vi "initUndo_Redo_stacks.vi"(8 "error in (no error)":errorcluster, 11 "ScriptEditorV2 in":refnum<class "ScriptEditorV2.lvclass">) -> (0 "error out":errorcluster, 3 "ScriptEditorV2 out":refnum<class "ScriptEditorV2.lvclass">)   [LabVIEW 2009, in "Views.lvlib" / "ScriptEditor.lvlib" / "ScriptEditorV2.lvclass"]
uses:
  ScriptEditorV2.lvclass
  ScriptEditorV2.lvclass/ScriptEditorV2.ctl
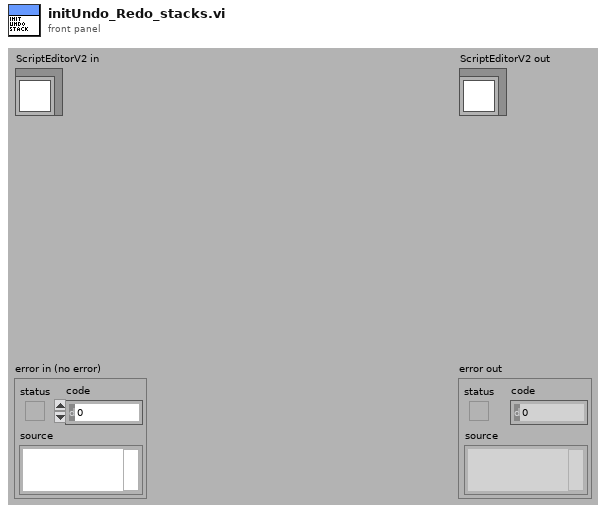
[diagram p1: front panel]
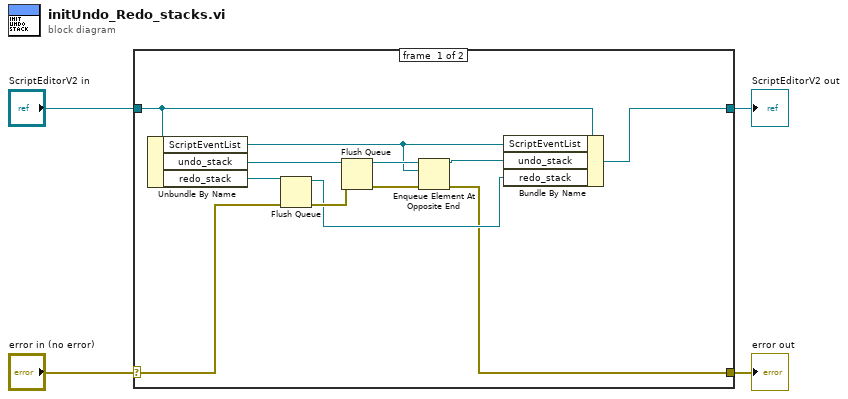
[diagram p0: block diagram]
diagram:
  n1 = case shown="No Error" "error in (no error)" {
    selector: "error in (no error)" -> [w13 w18]
    tunnel: [w5 w18] -> w3
    tunnel: [w6 w17] -> w1
    tunnel: "ScriptEditorV2 in" -> [w7 w17]
    frame #0 {
      n2 = Unbundle By Name(w7) -> ("ScriptEventList"=w10:refnum<class "ScriptEventList.lvclass">, "undo_stack"=w16:refnum<queue>, "redo_stack"=w14:refnum<queue>)
      n3 = Flush Queue(queue=w14, error in (no error)=w13) -> (queue out=w8:refnum<queue>, error out=w15:errorcluster)  [unwired: 1 out]
      n4 = Flush Queue(queue=w16, error in (no error)=w15) -> (queue out=w12:refnum<queue>, error out=w11:errorcluster)  [unwired: 1 out]
      n5 = Enqueue Element At Opposite End(queue=w12, element=w10, error in (no error)=w11) -> (queue out=w9:refnum<queue>, error out=w5:errorcluster)  [unwired: 1 in, 1 out]
      n6 = Bundle By Name(cluster=w7, "ScriptEventList"=w10, "undo_stack"=w9, "redo_stack"=w8) -> (w6:refnum<class "ScriptEditorV2.lvclass">)
    }
    frame #1 {
    }
  }
  "error out" <- w3
  "ScriptEditorV2 out" <- w1
